vi "ACQREF.vi"(7 "ACQ=1/REF=0":bool=TRUE, 8 "error in (no error)":errorcluster, 11 "VISA resource name":refnum<visa-resource-name>) -> (0 "100%":bool, 1 "75%":bool, 2 "50%":bool, 3 "25%":bool, 4 "error out":errorcluster, 5 "Number_array":u32[](array[numeric]))   [LabVIEW 2010]
uses:
  <vilib>/Instr/_visa.llb/VISA Configure Serial Port (Instr).vi
panel:
  out "size(s)":i32
  out "String_array":string[](array[string])
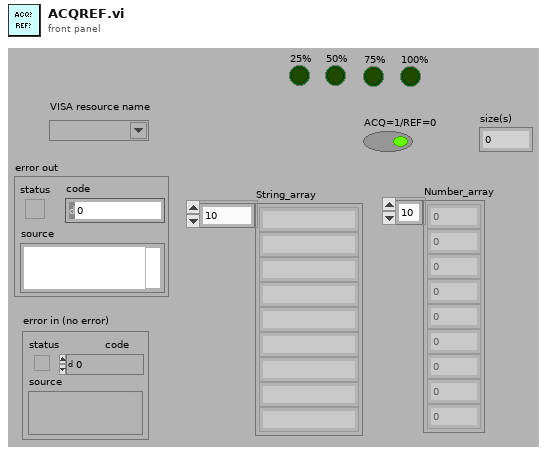
[diagram p1: front panel]
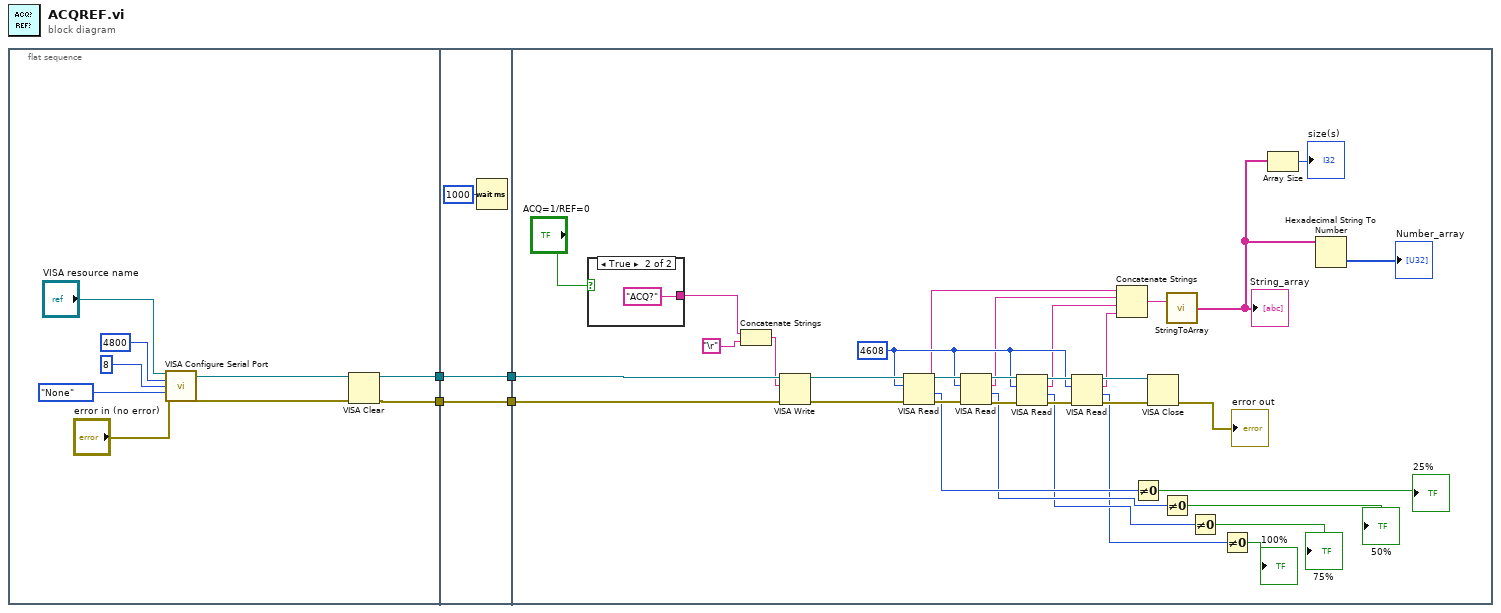
[diagram p0: block diagram]
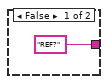
[diagram p2: hidden frame]
diagram:
  n1 = flat-sequence {
    tunnel: [w8] -> w2
    tunnel: [w7] -> w1
    tunnel: [w16] -> w4
    tunnel: [w15] -> w3
    tunnel: w2 -> [w16]
    tunnel: w1 -> [w15]
    tunnel: w4 -> [w47]
    tunnel: w3 -> [w46]
    frame #0 {
      n2 = call-poly "VISA Configure Serial Port"("VISA resource name"="VISA resource name", "baud rate (9600)"=u32 4800, "data bits (8)"=u16 8, "parity (0:none)"=enum16{"None", "Odd", "Even", "Mark", "Space"}."None", "error in (no error)"="error in (no error)") -> ("VISA resource name out"=w6:refnum<visa-resource-name>, "error out"=w5:errorcluster)  [unwired: 9 in]
      n3 = VISA Clear(VISA resource name=w6, error in (no error)=w5) -> (VISA resource name out=w8:refnum<visa-resource-name>, error out=w7:errorcluster)
    }
    frame #1 {
      n4 = Wait (ms)(milliseconds to wait=u32 1000) -> ()  [unwired: 1 out]
    }
    frame #2 {
      w39 = u32 4608 ("byte count")
      n5 = case shown="True" "ACQ=1/REF=0" {
        tunnel: ["REF?" ("string") "ACQ?" ("string")] -> w32
        frame False {
        }
        frame True {
        }
      }
      n6 = Concatenate Strings(w32, "\r") -> (w45:string)
      n7 = VISA Write(VISA resource name=w47, write buffer=w45, error in (no error)=w46) -> (VISA resource name out=w49:refnum<visa-resource-name>, error out=w50:errorcluster)  [unwired: 1 out]
      n8 = VISA Read(VISA resource name=w49, byte count=w39, error in (no error)=w50) -> (VISA resource name out=w43:refnum<visa-resource-name>, read buffer=w28:string, return count=w24:u32, error out=w38:errorcluster)
      n9 = VISA Read(VISA resource name=w43, byte count=w39, error in (no error)=w38) -> (VISA resource name out=w42:refnum<visa-resource-name>, read buffer=w27:string, return count=w23:u32, error out=w37:errorcluster)
      n10 = VISA Read(VISA resource name=w42, byte count=w39, error in (no error)=w37) -> (VISA resource name out=w41:refnum<visa-resource-name>, read buffer=w26:string, return count=w22:u32, error out=w36:errorcluster)
      n11 = VISA Read(VISA resource name=w41, byte count=w39, error in (no error)=w36) -> (VISA resource name out=w40:refnum<visa-resource-name>, read buffer=w25:string, return count=w21:u32, error out=w35:errorcluster)
      n12 = Concatenate Strings(w28, w27, w26, w25) -> (w34:string)
      n13 = Not Equal To 0?(x=w24) -> (x != 0?=→"25%":bool)
      n14 = VISA Close(VISA resource name=w40, error in (no error)=w35) -> (error out=→"error out":errorcluster)
      n15 = Not Equal To 0?(x=w23) -> (x != 0?=→"50%":bool)
      n16 = call "StringToArray.vi"("spreadsheet string"=w34) -> ("array"=w29:string[])
      "String_array" <- w29
      n17 = Not Equal To 0?(x=w22) -> (x != 0?=→"75%":bool)
      n18 = Not Equal To 0?(x=w21) -> (x != 0?=→"100%":bool)
      n19 = Array Size(array=w29) -> (size(s)=→"size(s)":i32)
      n20 = Hexadecimal String To Number(string=w29) -> (number=→"Number_array":u32[])  [unwired: 2 in, 1 out]
    }
  }
